vi "题目 4.vi"() -> ()   [LabVIEW 2017]
panel:
  in  "停止":bool
  in  "枚举":enum16{"王五", "李四", "张三"}(ring)
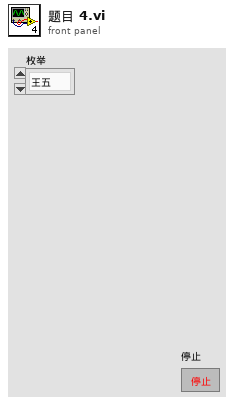
[diagram p1: front panel]
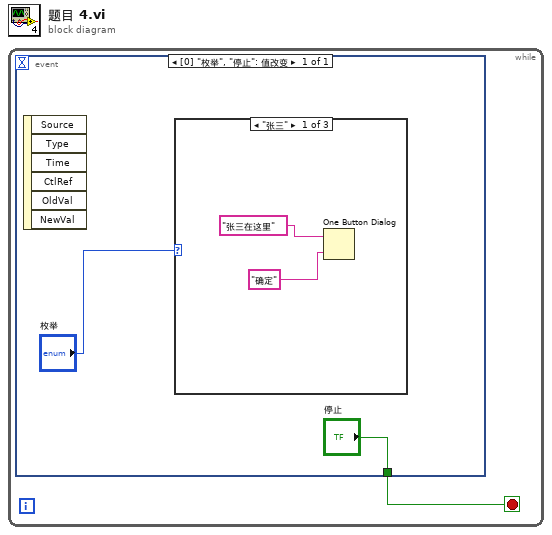
[diagram p0: block diagram]
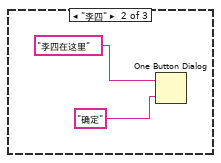
[diagram p2: hidden frame]
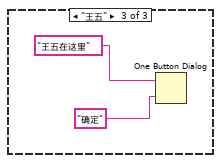
[diagram p3: hidden frame]
diagram:
  n1 = while {
    stop <- w1 stop-if-true
    n2 = event shown="[0] \"枚举\", \"停止\": 值改变" {
      selector: _ -> [_]
      dyn-events: _ -> [_]
      timeout: _ -> [_]
      tunnel: ["停止"] -> w1
      event "枚举", "停止": Value Change {
        n3 = event-data() -> ()  [unwired: 1 in, 6 out]
        n4 = case shown="\"张三\"" "枚举" {
          frame "张三" {
            n5 = One Button Dialog(message="张三在这里", button name ("OK")="确定") -> ()  [unwired: 1 out]
          }
          frame "李四" {
            n6 = One Button Dialog(message="李四在这里", button name ("OK")="确定") -> ()  [unwired: 1 out]
          }
          frame "王五" {
            n7 = One Button Dialog(message="王五在这里", button name ("OK")="确定") -> ()  [unwired: 1 out]
          }
        }
      }
    }
  }
